vi "XY Go.vi"(6 "return immediately":bool, 8 "error in (no error)":errorcluster, 9 "Speed":dbl, 10 "XY In":dbl[](array[numeric]), 11 "Gantry In":refnum<k24>) -> (0 "error out":errorcluster, 2 "XY Out 2":dbl[](array[numeric]), 3 "Gantry Out":refnum<k24>)   [LabVIEW 2018, in "Motion.lvclass"]
uses:
  Motion.lvclass
  C:/Program Files (x86)/Aerotech/A3200/LabVIEW/2010/Bin/Aerotech.A3200.dll
  Program Files (x86)/Aerotech/A3200/LabVIEW/2010/Bin/Aerotech.A3200.dll
  Drivers/Aerotech A3200/Aerotech.lvlib
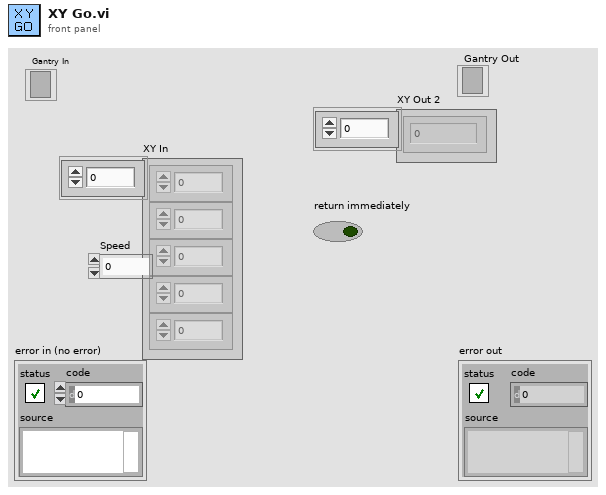
[diagram p1: front panel]
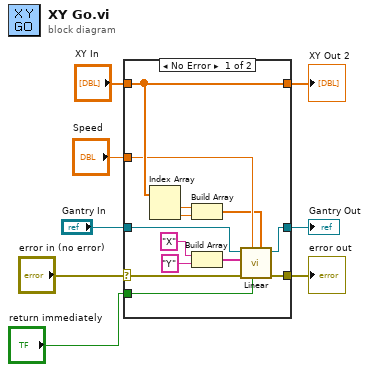
[diagram p0: block diagram]
diagram:
  n1 = case shown="No Error" "error in (no error)" {
    selector: "error in (no error)" -> [w9 w24]
    tunnel: [w10 w24] -> w7
    tunnel: "Gantry In" -> [w16 w23]
    tunnel: "XY In" -> [w17 w22]
    tunnel: "Speed" -> [w15 _]
    tunnel: [w11 w23] -> w3
    tunnel: [w17 w22] -> w2
    tunnel: "return immediately" -> [w12 _]
    frame No Error {
      n2 = Index Array(array=w17) -> (element #1=w19:dbl, element #2=w18:dbl)  [unwired: 2 in]
      n3 = Build Array(w19, w18) -> (w14:dbl[])
      n4 = Build Array("X" ("format string"), "Y" ("format string")) -> (w13:string[])
      n5 = call "Linear.vi"("distances"=w14, "return immediately"=w12, "speed"=w15, "error in (no error)"=w9, "axis names"=w13, "controller in"=w16) -> ("error out"=w10:errorcluster, "controller out"=w11:refnum<k24>)  [unwired: 4 in]
    }
    frame Error {
    }
  }
  "error out" <- w7
  "Gantry Out" <- w3
  "XY Out 2" <- w2
